vi "HTML Report Table.vi"(4 "Show Grid":bool, 5 "width":string, 6 "align (default)":T1, 7 "table rows":string, 8 "HTML in":string) -> (3 "HTML out":string)   [LabVIEW 2017, in "NI_ReportGenerationCore.lvlib"]
doc: "Constructs tags for an HTML table <TABLE> with the specified caption and table contents."
uses:
  <vilib>/Utility/NIReport.llb/NI_ReportGenerationCore.lvlib
  <vilib>/Utility/NIReport.llb/HTML Report Text Alignment.ctl
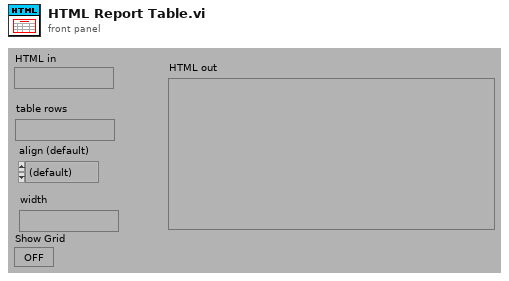
[diagram p1: front panel]
types:
  T1 = typedef "NI_ReportGenerationCore.lvlib/HTML Report Text Alignment.ctl" = enum16{"(default)", "LEFT", "CENTER", "RIGHT"}
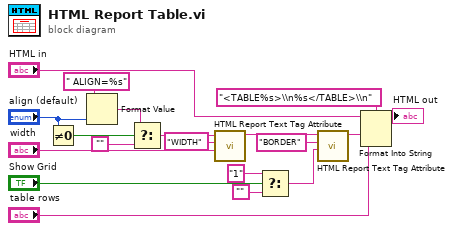
[diagram p0: block diagram]
diagram:
  n1 = Not Equal To 0?(x="align (default)") -> (x != 0?=w16:bool)
  n2 = Format Value(format string=" ALIGN=%s", value (0)="align (default)") -> (output string=w17:string)  [unwired: 1 out]
  n3 = Select(t=w17, s=w16, f="" ("Empty String Constant")) -> (s? t:f=w14:string)
  n4 = call <vilib>:"HTML Report Text Tag Attribute.vi"("value"="width", "label"="WIDTH" ("format string"), "tag attributes in"=w14) -> ("tag attributes out"=w6:string)  [unwired: 1 in, 3 out]
  n5 = Select(t="1", s="Show Grid", f="" ("Empty String Constant")) -> (s? t:f=w2:string)
  n6 = call <vilib>:"HTML Report Text Tag Attribute.vi"("value"=w2, "label"="BORDER", "tag attributes in"=w6) -> ("tag attributes out"=w7:string)  [unwired: 1 in, 3 out]
  n7 = Format Into String(format string="<TABLE%s>\\n%s</TABLE>\\n", initial string="HTML in", w7, "table rows") -> (resulting string=→"HTML out":string)  [unwired: 1 in, 1 out]
